vi "RPS to Rev.vi"(1 "rad/s":dbl) -> (0 "rpm":i64)   [LabVIEW 2019]
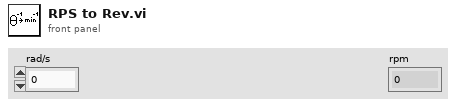
[diagram p1: front panel]
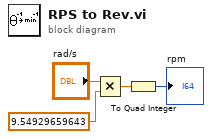
[diagram p0: block diagram]
diagram:
  n1 = Multiply(x="rad/s", y=9.54929659643) -> (x*y=w2:dbl)
  n2 = To Quad Integer(1:w2) -> (0:→"rpm":i64)
